vi "add scan time(SubVI).vi"(10 "字符串":string) -> (1 "ok or cancel":bool, 2 "连接的字符串":string)   [LabVIEW 2019, in "Add Seq.lvlib"]
uses:
  Add Seq.lvlib
panel:
  in  "steps":i32
  in  "total time":dbl
  in  "cancel":bool
  in  "ok":bool
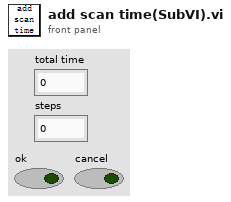
[diagram p1: front panel]
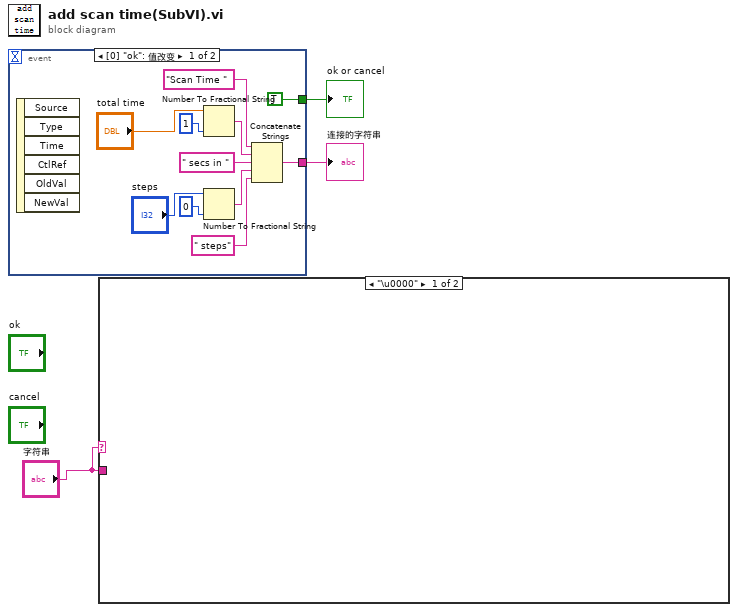
[diagram p0: block diagram]
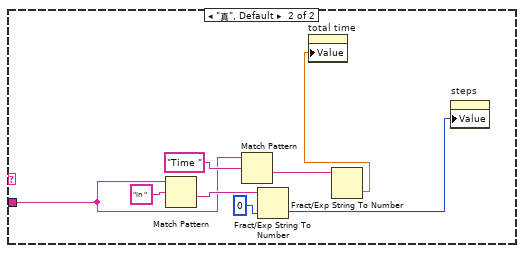
[diagram p2: hidden frame]
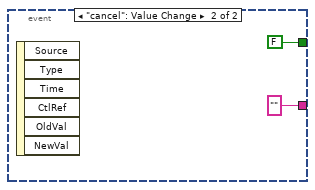
[diagram p3: hidden frame]
diagram:
  n1 = event shown="[0] \"ok\": 值改变" {
    selector: _ -> [_ _]
    dyn-events: _ -> [_ _]
    timeout: _ -> [_ _]
    tunnel: [TRUE FALSE] -> w3
    tunnel: [w4 "" ("分隔符")] -> w2
    event "ok": Value Change {
      n2 = event-data() -> ()  [unwired: 1 in, 6 out]
      n3 = Number To Fractional String(number="total time", precision (6)=i16 1 ("精度(6)")) -> (F-format string=w11:string)  [unwired: 2 in]
      n4 = Number To Fractional String(number="steps", precision (6)=i16 0 ("精度(6)")) -> (F-format string=w6:string)  [unwired: 2 in]
      n5 = Concatenate Strings("Scan Time " ("字符串"), w11, " secs in " ("字符串"), w6, " steps" ("字符串")) -> (w4:string)
    }
    event "cancel": Value Change {
      n6 = event-data() -> ()  [unwired: 1 in, 6 out]
    }
  }
  "ok or cancel" <- w3
  "连接的字符串" <- w2
  n7 = case shown="\"\"" "字符串" {
    tunnel: "字符串" -> [_ w19]
    frame "\u0000" {
    }
    frame "真", Default {
      n8 = Match Pattern(string=w19, regular expression="in " ("正则表达式")) -> (after substring=w21:string)  [unwired: 1 in, 3 out]
      n9 = Match Pattern(string=w19, regular expression="Time " ("正则表达式")) -> (after substring=w23:string)  [unwired: 1 in, 3 out]
      n10 = Fract/Exp String To Number(string=w21, default (0 dbl)=0) -> (number=w18:i32)  [unwired: 2 in, 1 out]
      n11 = Fract/Exp String To Number(string=w23) -> (number=w17:dbl)  [unwired: 3 in, 1 out]
      n12 = property on="total time" class="DigNum (严格)"("Value"=w17) -> ()  [unwired: 2 in, 2 out]
      n13 = property on="steps" class="DigNum (严格)"("Value"=w18) -> ()  [unwired: 2 in, 2 out]
    }
  }
